vi "Clear pretomo IMAQ.vi"(8 "error in (no error)":errorcluster, 11 "Tomo in":refnum<class "Tomo.lvclass">) -> (0 "error out":errorcluster, 3 "Tomo out":refnum<class "Tomo.lvclass">)   [LabVIEW 2012, in "Tomo.lvclass"]
uses:
  Tomo.lvclass
  Tomo.lvclass/Tomo.ctl
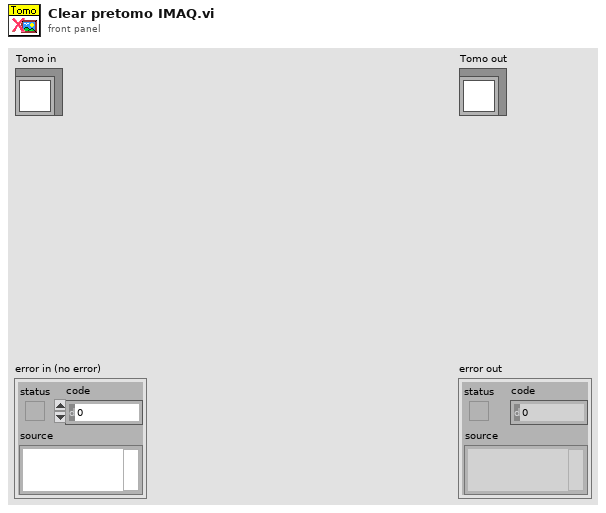
[diagram p1: front panel]
types:
  T1 = typedef "IMAQ Image.ctl" = refnum<image>
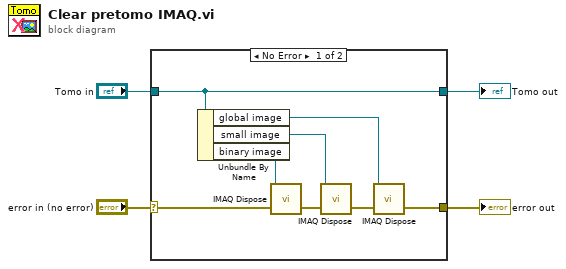
[diagram p0: block diagram]
diagram:
  n1 = case shown="No Error" "error in (no error)" {
    selector: "error in (no error)" -> [w9 w14]
    tunnel: [w8 w14] -> w3
    tunnel: [w12 w13] -> w1
    tunnel: "Tomo in" -> [w12 w13]
    frame No Error {
      n2 = Unbundle By Name(w12) -> ("global image"=w5:T1, "small image"=w6:T1, "binary image"=w7:T1)
      n3 = call "IMAQ Dispose"("Image"=w7, "error in (no error)"=w9) -> ("error out"=w11:errorcluster)  [unwired: 4 in]
      n4 = call "IMAQ Dispose"("Image"=w6, "error in (no error)"=w11) -> ("error out"=w10:errorcluster)  [unwired: 4 in]
      n5 = call "IMAQ Dispose"("Image"=w5, "error in (no error)"=w10) -> ("error out"=w8:errorcluster)  [unwired: 4 in]
    }
    frame Error {
    }
  }
  "error out" <- w3
  "Tomo out" <- w1
